vi "日期时间对话框.vi"(7 "first":i32 caption="第一", 8 "wdnames":string[](array[string])=["日", "一", "二", "三", "四", "五", "六"] caption="星期名称", 9 "fmtstr":string="%<%.3X\n%x>T" caption="格式字符串", 10 "secin":timestamp caption="秒输入", 11 "mnames":string[](array[string])=["一月", "二月", "三月", "四月", "五月", "六月", "七月", "八月", "九月", "十月", "十一月", "十二月"] caption="月份名称") -> (1 "ok":bool caption="确定", 2 "secout":timestamp caption="秒输出" format="%<%Z>T")   [LabVIEW 2011]
panel:
  in  "help":bool caption="取消"
  out "DaylightSavingState":string caption="夏令时状态"
  out "date time rec":T1 caption="日期时间记录"
  in  "Time Display":timestamp caption="时间显示" format="%<%.3X>T"
  in  "now":bool caption="现在"
  in  "cancel":bool caption="取消"
  in  "ok":bool caption="确定"
  in  "Year":i32=1905 caption="年" min=1600 max=3000
  in  "Month":i32(ring) caption="月" items=["一月", "二月", "三月", "四月", "五月", "六月", "七月", "八月", "九月", "十月", "十一月", "十二月"]
  in  "Date":i32(listbox) caption="日期"
  # "（0表示星期天，1表示星期一，等）"
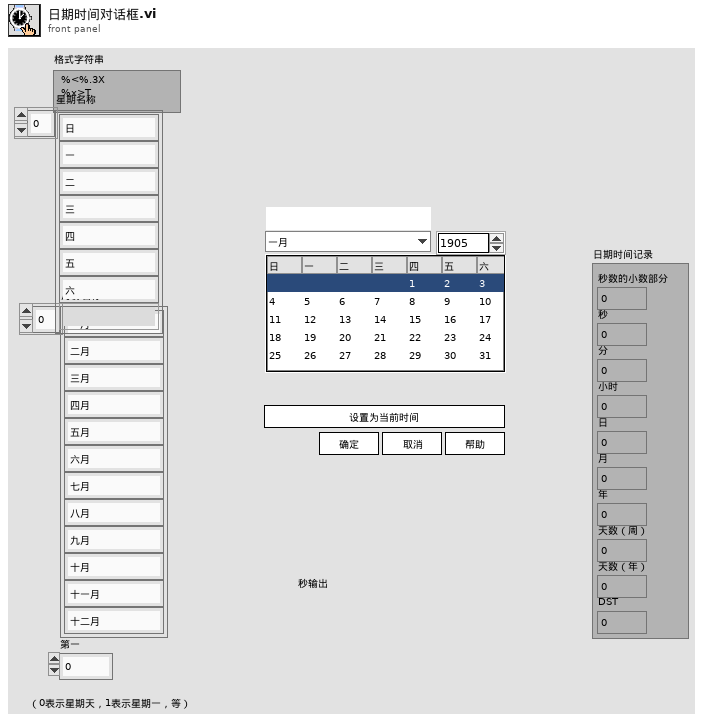
[diagram p1: front panel]
types:
  T1 = cluster{"fractional second":dbl, "second":i32, "minute":i32, "hour":i32, "day of month":i32, "month":i32, "year":i32, "day of week":i32, "day of year":i32, "DST":i32}
  T2 = typedef "LVDateTimeRec.ctl" = cluster{"fractional second":dbl, "second":i32, "minute":i32, "hour":i32, "day of month":i32, "month":i32, "year":i32, "day of week":i32, "day of year":i32, "DST":i32}
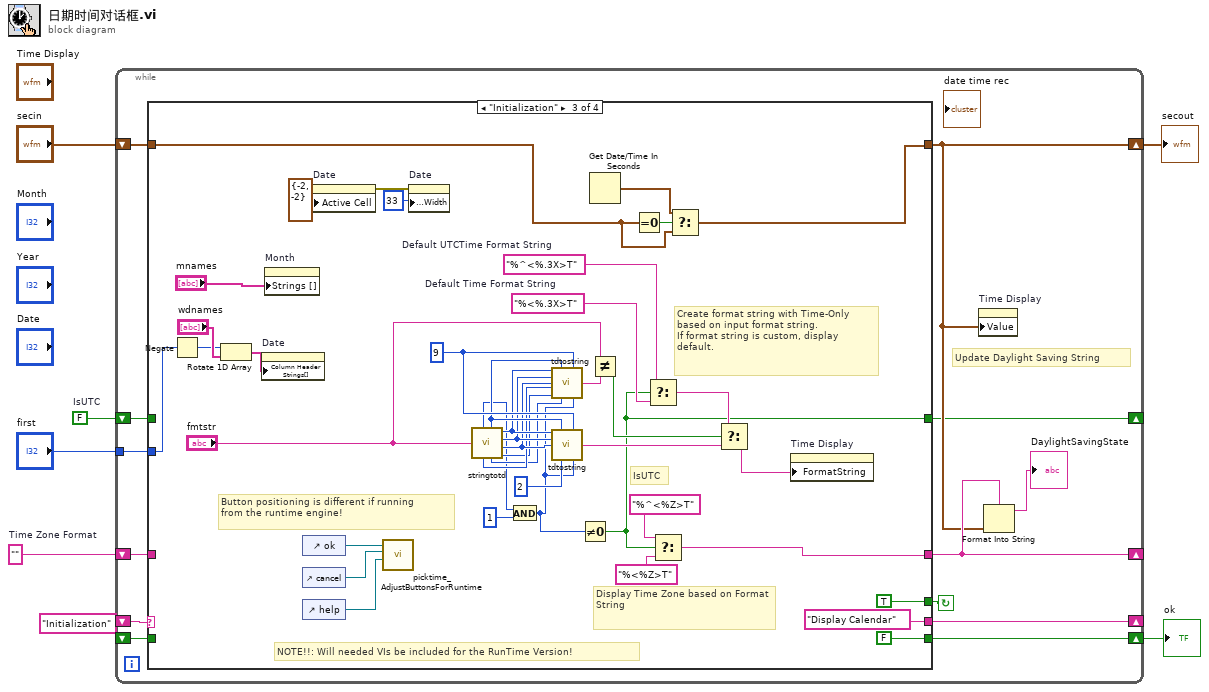
[diagram p0: block diagram]
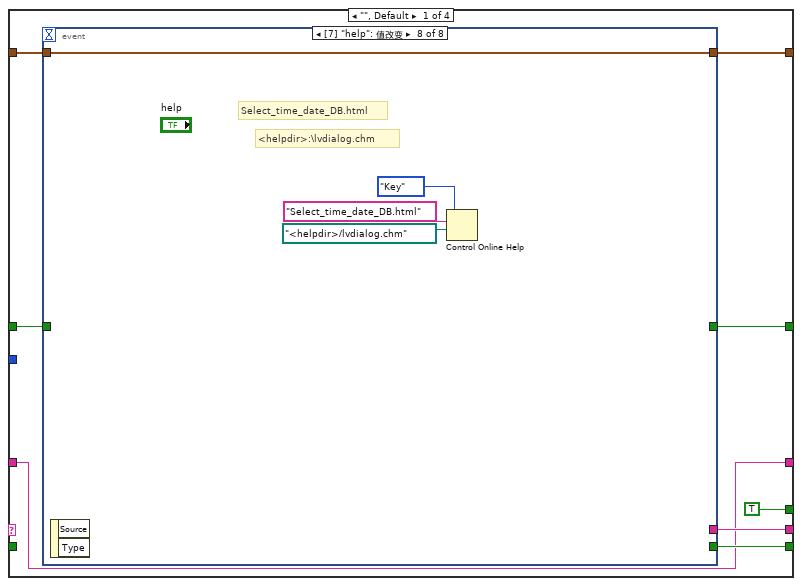
[diagram p2: hidden frame]
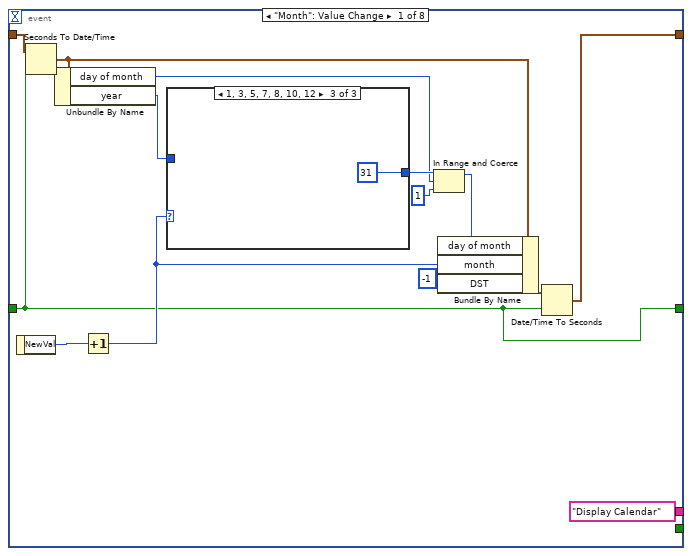
[diagram p3: hidden frame]
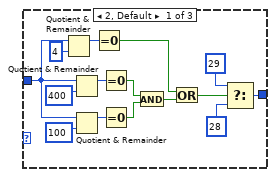
[diagram p4: hidden frame]
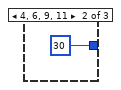
[diagram p5: hidden frame]
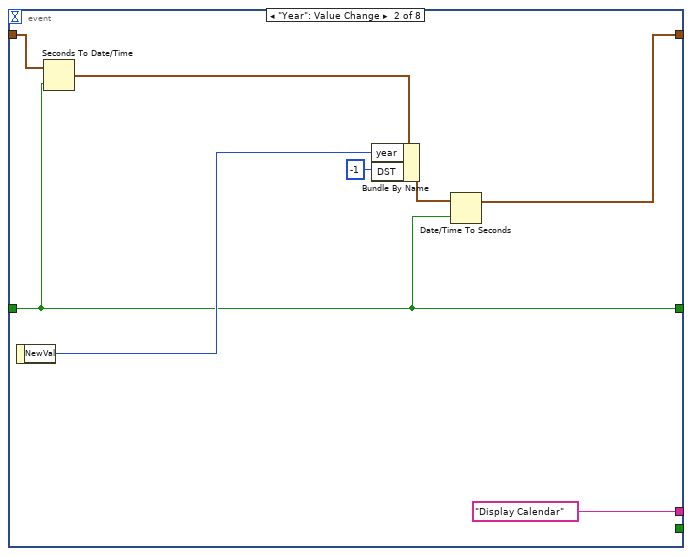
[diagram p6: hidden frame]
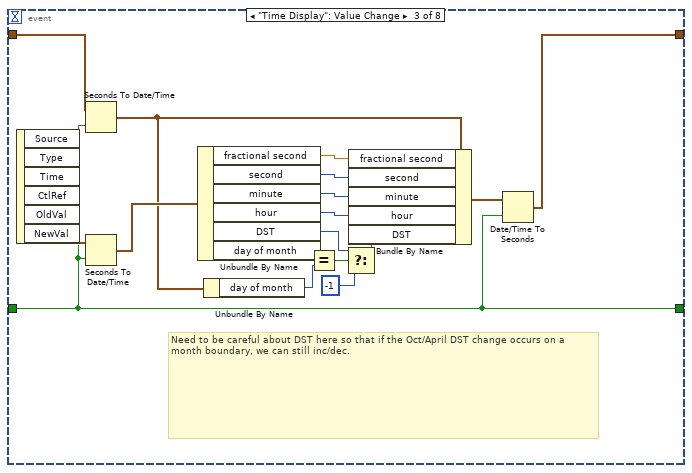
[diagram p7: hidden frame]
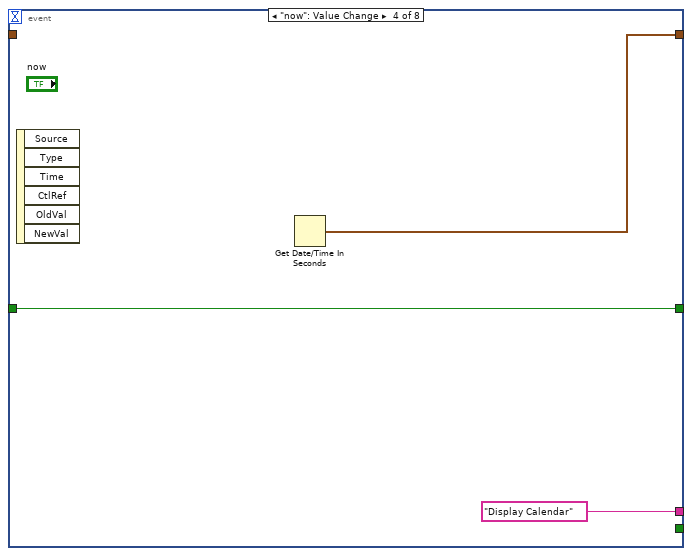
[diagram p8: hidden frame]
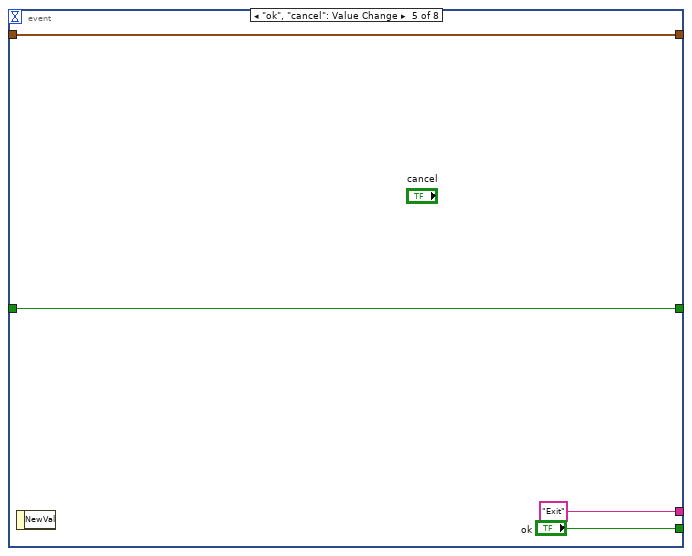
[diagram p9: hidden frame]
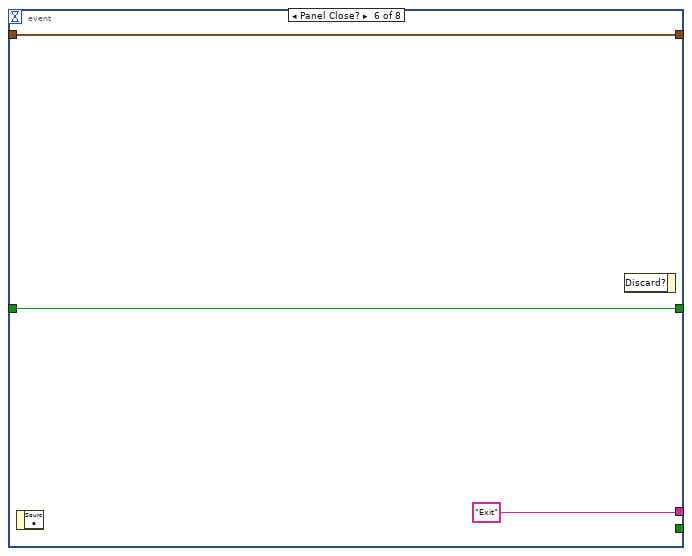
[diagram p10: hidden frame]
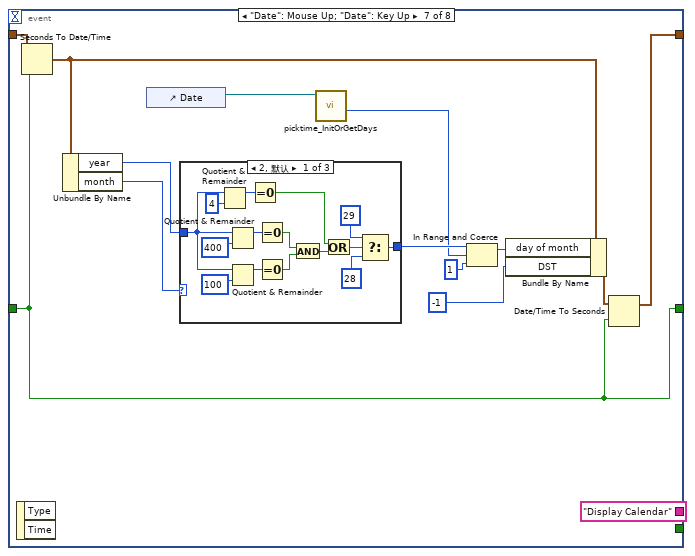
[diagram p11: hidden frame]
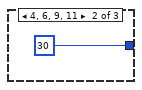
[diagram p12: hidden frame]
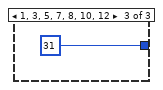
[diagram p13: hidden frame]
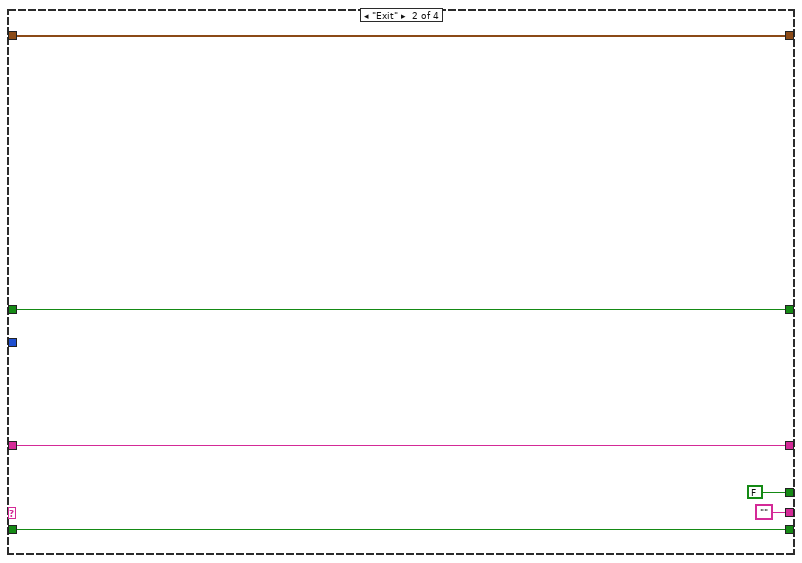
[diagram p14: hidden frame]
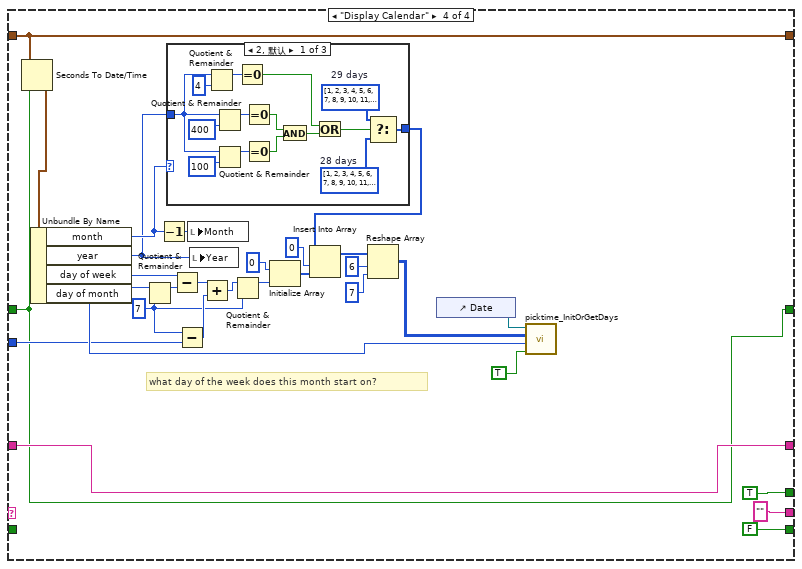
[diagram p15: hidden frame]
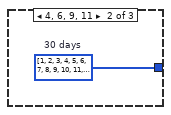
[diagram p16: hidden frame]
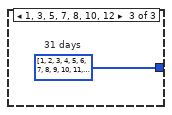
[diagram p17: hidden frame]
diagram:
  w1 = FALSE  # IsUTC
  w3 = ""  # Time Zone Format
  n1 = while {
    shift-right: [w19] -> _
    shift-left: "Initialization" -> [w20]
    shift-right: [w11] -> w4
    shift-left: "secin" -> [w18]
    shift-right: [w16] -> w6
    shift-left: _ -> [w15]
    shift-right: [w12] -> _
    shift-left: w3 -> [w14]
    tunnel: "first" -> [w10]
    shift-right: [w8] -> _
    shift-left: w1 -> [w9]
    stop <- w17 continue-if-true
    # "Update Daylight Saving String"
    n2 = case shown="\"Initialization\"" w20 {
      tunnel: [w25 "" "Display Calendar" ""] -> w19
      tunnel: [TRUE FALSE TRUE TRUE] -> w17
      tunnel: w18 -> [w26 w132 w168 w188]
      tunnel: [w27 w132 w167 w188] -> w11
      tunnel: [w24 w133 FALSE ("ok") FALSE ("ok")] -> w16
      tunnel: w15 -> [_ w133 _ _]
      tunnel: [w23 w131 w147 w187] -> w12
      tunnel: w14 -> [w23 w131 _ w187]
      tunnel: w10 -> [_ _ w143 w183]
      tunnel: w9 -> [w22 w130 _ w180]
      tunnel: [w21 w130 w141 w180] -> w8
      frame "", Default {
        n3 = event shown="[7] \"help\": 值改变" {
          selector: _ -> [_ _ _ _ _ _ _ _]
          dyn-events: _ -> [_ _ _ _ _ _ _ _]
          timeout: _ -> [_ _ _ _ _ _ _ _]
          tunnel: w26 -> [w32 w63 w83 _ w89 w93 w100 w129]
          tunnel: [w31 w61 w81 w86 w89 w93 w98 w129] -> w27
          tunnel: ["Display Calendar" "Display Calendar" _ "Display Calendar" "Exit" "Exit" "Display Calendar" _] -> w25
          tunnel: [_ _ _ _ "ok" _ _ _] -> w24
          tunnel: w22 -> [w29 w60 w68 w85 w88 w92 w97 _]
          tunnel: [w29 w60 w68 w85 w88 w92 w97 _] -> w21
          event "Month": Value Change {
            n4 = event-data() -> ("NewVal"=w42:i32)  [unwired: 1 out]
            n5 = Seconds To Date/Time(time stamp (now)=w32, to UTC (F)=w29) -> (date time rec=w30:T2)
            n6 = Unbundle By Name(w30) -> ("day of month"=w36:i32, "year"=w37:i32)
            n7 = Increment(x=w42) -> (x+1=w40:i32)
            n8 = case shown="1, 3, 5, 7, 8, 10, 12" w40 {
              tunnel: [w55 30 31] -> w39
              tunnel: w37 -> [w50 _ _]
              frame 2, Default {
                n9 = Quotient & Remainder(x=w50, y=4) -> (x-y*floor(x/y)=w54:i32)  [unwired: 1 out]
                n10 = Quotient & Remainder(x=w50, y=400) -> (x-y*floor(x/y)=w49:i32)  [unwired: 1 out]
                n11 = Quotient & Remainder(x=w50, y=100) -> (x-y*floor(x/y)=w48:i32)  [unwired: 1 out]
                n12 = Equal To 0?(x=w54) -> (x = 0?=w53:bool)
                n13 = Equal To 0?(x=w49) -> (x = 0?=w46:bool)
                n14 = Equal To 0?(x=w48) -> (x = 0?=w47:bool)
                n15 = And(x=w46, y=w47) -> (x .and. y?=w45:bool)
                n16 = Or(x=w53, y=w45) -> (x .or. y?=w52:bool)
                n17 = Select(t=29, s=w52, f=28) -> (s? t:f=w55:i32)
              }
              frame 4, 6, 9, 11 {
              }
              frame 1, 3, 5, 7, 8, 10, 12 {
              }
            }
            n18 = In Range and Coerce(upper limit=w39, x=w36, lower limit=1) -> (coerced(x)=w35:i32)  [unwired: 1 out]
            n19 = Bundle By Name(cluster=w30, "day of month"=w35, "month"=w40, "DST"=-1) -> (w34:T2)
            n20 = Date/Time To Seconds(1:w29, 2:w34) -> (0:w31:timestamp)
          }
          event "Year": Value Change {
            n21 = event-data() -> ("NewVal"=w67:i32)  [unwired: 1 out]
            n22 = Seconds To Date/Time(time stamp (now)=w63, to UTC (F)=w60) -> (date time rec=w62:T2)
            n23 = Bundle By Name(cluster=w62, "year"=w67, "DST"=-1) -> (w65:T2)
            n24 = Date/Time To Seconds(1:w60, 2:w65) -> (0:w61:timestamp)
          }
          event "Time Display": Value Change {
            # "Need to be careful about DST here so that if the Oct/April DST change occurs on a month boundary, we can still inc/dec."
            n25 = event-data() -> ("NewVal"=w84:timestamp)  [unwired: 6 out]
            n26 = Seconds To Date/Time(time stamp (now)=w83, to UTC (F)=w68) -> (date time rec=w71:T2)
            n27 = Seconds To Date/Time(time stamp (now)=w84, to UTC (F)=w68) -> (date time rec=w80:T2)
            n28 = Unbundle By Name(w80) -> ("fractional second"=w76:dbl, "second"=w77:i32, "minute"=w78:i32, "hour"=w79:i32, "DST"=w73:i32, "day of month"=w69:i32)
            n29 = Unbundle By Name(w71) -> ("day of month"=w70:i32)
            n30 = Equal?(x=w69, y=w70) -> (x = y?=w75:bool)
            n31 = Select(t=w73, s=w75, f=-1) -> (s? t:f=w72:i32)
            n32 = Bundle By Name(cluster=w71, "fractional second"=w76, "second"=w77, "minute"=w78, "hour"=w79, "DST"=w72) -> (w82:T2)
            n33 = Date/Time To Seconds(1:w68, 2:w82) -> (0:w81:timestamp)
          }
          event "now": Value Change {
            n34 = event-data() -> ()  [unwired: 7 out]
            n35 = Get Date/Time In Seconds() -> (seconds since 1Jan1904=w86:timestamp)
          }
          event "ok", "cancel": Value Change {
            n36 = event-data() -> ()  [unwired: 2 out]
          }
          event Panel Close? {
            n37 = event-data() -> ()  [unwired: 2 out]
            n38 = event-data() -> ()  [unwired: 1 in, 2 out]
          }
          event "Date": Mouse Up; "Date": Key Up {
            n39 = event-data() -> ()  [unwired: 3 out]
            n40 = Seconds To Date/Time(time stamp (now)=w100, to UTC (F)=w97) -> (date time rec=w99:T2)
            n41 = Unbundle By Name(w99) -> ("year"=w106:i32, "month"=w105:i32)
            n42 = control-ref of="Date"() -> (w95:refnum<vi>)
            n43 = case shown="2, 默认" w105 {
              tunnel: [w121 30 31] -> w108
              tunnel: w106 -> [w116 _ _]
              frame 2, Default {
                n44 = Quotient & Remainder(x=w116, y=4) -> (x-y*floor(x/y)=w120:i32)  [unwired: 1 out]
                n45 = Quotient & Remainder(x=w116, y=400) -> (x-y*floor(x/y)=w115:i32)  [unwired: 1 out]
                n46 = Quotient & Remainder(x=w116, y=100) -> (x-y*floor(x/y)=w114:i32)  [unwired: 1 out]
                n47 = Equal To 0?(x=w120) -> (x = 0?=w119:bool)
                n48 = Equal To 0?(x=w115) -> (x = 0?=w112:bool)
                n49 = Equal To 0?(x=w114) -> (x = 0?=w113:bool)
                n50 = And(x=w112, y=w113) -> (x .and. y?=w111:bool)
                n51 = Or(x=w119, y=w111) -> (x .or. y?=w118:bool)
                n52 = Select(t=29, s=w118, f=28) -> (s? t:f=w121:i32)
              }
              frame 4, 6, 9, 11 {
              }
              frame 1, 3, 5, 7, 8, 10, 12 {
              }
            }
            n53 = call "picktime_InitOrGetDays.vi"("reference"=w95) -> ("day of month(out)"=w96:i32)  [unwired: 3 in, 7 out]
            n54 = In Range and Coerce(upper limit=w108, x=w96, lower limit=1) -> (coerced(x)=w104:i32)  [unwired: 1 out]
            n55 = Bundle By Name(cluster=w99, "day of month"=w104, "DST"=-1) -> (w102:T2)
            n56 = Date/Time To Seconds(1:w97, 2:w102) -> (0:w98:timestamp)
          }
          event "help": Value Change {
            # "<helpdir>:\\lvdialog.chm"
            # "Select_time_date_DB.html"
            n57 = event-data() -> ()  [unwired: 3 out]
            n58 = Control Online Help(2:path "<helpdir>/lvdialog.chm" ("Path to the help file"), 3:"Select_time_date_DB.html" ("String to search for"), 4:enum16{"Contents", "Key", "Close"}."Key" ("Operation")) -> ()  [unwired: 1 in, 1 out]
          }
        }
      }
      frame "Exit" {
      }
      frame "Initialization" {
        w150 = "%^<%.3X>T"  # Default UTCTime Format String
        w149 = "%<%.3X>T"  # Default Time Format String
        w163 = 9 ("Type (9 = Absolute)")
        # "Button positioning is different if running\nfrom the runtime engine!"
        # "IsUTC"
        # "Display Time Zone based on Format String"
        # "NOTE!!: Will needed VIs be included for the RunTime Version!"
        # "Create format string with Time-Only based on input format string.\nIf format string is custom, display default."
        n59 = Negate(x=w143) -> (-x=w142:i32)
        n60 = Rotate 1D Array(1:"wdnames", 2:w142) -> (0:w145:string[])
        n61 = property on="Date" class="MCListbox (严格)"("Column Header Strings[]"=w145) -> ()  [unwired: 2 in, 2 out]
        n62 = property on="Month" class="Ring (严格)"("Strings []"="mnames") -> ()  [unwired: 2 in, 2 out]
        n63 = control-ref of="ok"() -> (w138:refnum<vi>)
        n64 = control-ref of="cancel"() -> (w137:refnum<vi>)
        n65 = control-ref of="help"() -> (w136:refnum<vi>)
        n66 = property on="Date" class="MCListbox (严格)"("Active Cell"=cluster{i32, i32} {-2, -2}) -> (error out=w175:errorcluster)  [unwired: 2 in, 1 out]
        n67 = call "picktime_AdjustButtonsForRuntime.vi"("help button ref"=w136, "cancel button ref"=w137, "ok button ref"=w138) -> ()  [unwired: 9 out]
        n68 = property on="Date" class="MCListbox (严格)"(error in=w175, "Cell Size:Width"=u32 33) -> ()  [unwired: 1 in, 2 out]
        n69 = call "stringtotd.vi"("Time & Date Format String"="fmtstr") -> ("UTC"=w139:i16, "MDY"=w158:i16, "Time Format"=w162:i16, "AM/PM"=w161:i16, "included seconds"=w160:i16, "Date Format"=w156:i16, "seconds precision"=w159:i16, "Year Format"=w157:i16)  [unwired: 2 out]
        n70 = And(x=w139, y=i16 1) -> (x .and. y?=w140:i16)
        n71 = call "tdtostring.vi"("AM/PM"=w161, "Time Format"=w162, "Type (10 = Absolute)"=w163, "included seconds"=w160, "seconds precision"=w159, "m-d-y sequence"=w158, "year format"=w157, "Date Format"=w156, "UTC"=w140) -> ("Format String"=w154:string)  [unwired: 2 in, 4 out]
        n72 = call "tdtostring.vi"("AM/PM"=w161, "Time Format"=w162, "Type (10 = Absolute)"=w163, "included seconds"=w160, "seconds precision"=w159, "Date Format"=i16 2, "UTC"=w140) -> ("Format String"=w152:string)  [unwired: 4 in, 4 out]
        n73 = Not Equal To 0?(x=w140) -> (x != 0?=w141:bool)
        n74 = Get Date/Time In Seconds() -> (seconds since 1Jan1904=w170:timestamp)
        n75 = Not Equal?(x="fmtstr", y=w154) -> (x != y?=w153:bool)
        n76 = Equal To 0?(x=w168) -> (x = 0?=w171:bool)
        n77 = Select(t=w150, s=w141, f=w149) -> (s? t:f=w148:string)
        n78 = Select(t="%^<%Z>T", s=w141, f="%<%Z>T") -> (s? t:f=w147:string)
        n79 = Select(t=w170, s=w171, f=w168) -> (s? t:f=w167:timestamp)
        n80 = Select(t=w148, s=w153, f=w152) -> (s? t:f=w151:string)
        n81 = property on="Time Display" class="AbsTime (严格)"("FormatString"=w151) -> ()  [unwired: 2 in, 2 out]
      }
      frame "Display Calendar" {
        w181 = 7 ("y")
        # "what day of the week does this month start on?"
        n82 = Seconds To Date/Time(time stamp (now)=w188, to UTC (F)=w180) -> (date time rec=w189:T2)
        n83 = Unbundle By Name(w189) -> ("month"=w195:i32, "year"=w194:i32, "day of week"=w205:i32, "day of month"=w186:i32)
        n84 = Quotient & Remainder(x=w186, y=w181) -> (x-y*floor(x/y)=w204:i32)  [unwired: 1 out]
        n85 = Decrement(x=w195) -> (x-1=w196:i32)
        n86 = case shown="2, 默认" w195 {
          tunnel: [w219 w222 w223] -> w190
          tunnel: w194 -> [w212 _ _]
          frame 2, Default {
            w217 = i32[] [1, 2, 3, 4, 5, 6, 7, 8, 9, 10, 11, 12, 13, 14, 15, 16, 17, 18, 19, 20, 21, 22, 23, 24, 25, 26, 27, 28]  # 28 days
            w218 = i32[] [1, 2, 3, 4, 5, 6, 7, 8, 9, 10, 11, 12, 13, 14, 15, 16, 17, 18, 19, 20, 21, 22, 23, 24, 25, 26, 27, 28, 29]  # 29 days
            n87 = Quotient & Remainder(x=w212, y=4) -> (x-y*floor(x/y)=w216:i32)  [unwired: 1 out]
            n88 = Quotient & Remainder(x=w212, y=400) -> (x-y*floor(x/y)=w211:i32)  [unwired: 1 out]
            n89 = Quotient & Remainder(x=w212, y=100) -> (x-y*floor(x/y)=w210:i32)  [unwired: 1 out]
            n90 = Equal To 0?(x=w216) -> (x = 0?=w215:bool)
            n91 = Equal To 0?(x=w211) -> (x = 0?=w208:bool)
            n92 = Equal To 0?(x=w210) -> (x = 0?=w209:bool)
            n93 = And(x=w208, y=w209) -> (x .and. y?=w207:bool)
            n94 = Or(x=w215, y=w207) -> (x .or. y?=w214:bool)
            n95 = Select(t=w218, s=w214, f=w217) -> (s? t:f=w219:i32[])
          }
          frame 4, 6, 9, 11 {
            w222 = i32[] [1, 2, 3, 4, 5, 6, 7, 8, 9, 10, 11, 12, 13, 14, 15, 16, 17, 18, 19, 20, 21, 22, 23, 24, 25, 26, 27, 28, 29, 30]  # 30 days
          }
          frame 1, 3, 5, 7, 8, 10, 12 {
            w223 = i32[] [1, 2, 3, 4, 5, 6, 7, 8, 9, 10, 11, 12, 13, 14, 15, 16, 17, 18, 19, 20, 21, 22, 23, 24, 25, 26, 27, 28, 29, 30, 31]  # 31 days
          }
        }
        n96 = Subtract(x=w205, y=w204) -> (x-y=w185:i32)
        n97 = Subtract(x=w181, y=w183) -> (x-y=w182:i32)
        n98 = local write "Month"(w196) -> ()
        n99 = local write "Year"(w194) -> ()
        n100 = Add(x=w185, y=w182) -> (x+y=w184:i32)
        n101 = Quotient & Remainder(x=w184, y=w181) -> (x-y*floor(x/y)=w193:i32)  [unwired: 1 out]
        n102 = Initialize Array(0, w193) -> (w201:i32[])
        n103 = Insert Into Array(array=w190, index=0, new element=w201) -> (w199:i32[])
        n104 = Reshape Array(w199, 6 ("dimension size"), 7 ("dimension size")) -> (w192:i32[][])
        n105 = control-ref of="Date"() -> (w179:refnum<vi>)
        n106 = call "picktime_InitOrGetDays.vi"("Init"=TRUE, "day of month"=w186, "31 days"=w192, "reference"=w179) -> ()  [unwired: 8 out]
      }
    }
    n107 = property on="Time Display" class="AbsTime (严格)"("Value"=w11) -> ()  [unwired: 2 in, 2 out]
    n108 = Format Into String(format string=w12, w11) -> (resulting string=→"DaylightSavingState":string)  [unwired: 2 in, 1 out]
  }
  "ok" <- w6
  "secout" <- w4
